vi "Discrete Limited Integrator.vi"   [LabVIEW 2017, in "NI_AdvCtrl_discrete linear.lvlib"]
doc: "LabVIEW no longer supports this VI. You can obtain similar functionality by installing the LabVIEW Simulation Module.\n\nIntegrates a discrete input signal. The result of the discrete integration is limited by the lower and upper bound."
uses:
  <vilib>/addons/control/advanced/NI_AdvCtrl_discrete linear.lvlib
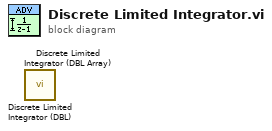
[diagram p0: block diagram]
diagram:
  n1 = call <vilib>:"Discrete Limited Integrator (DBL).vi"() -> ()  [unwired: 6 in, 1 out]
  n2 = call <vilib>:"Discrete Limited Integrator (DBL Array).vi"() -> ()  [unwired: 6 in, 1 out]
